vi "sub_vi_get_linear_parameters.vi"(8 "error in":errorcluster, 11 "VISA resource name in":refnum<visa-resource-name>) -> (0 "error out":errorcluster, 1 "intercept_2":dbl, 2 "slope_2":dbl, 3 "VISA resource name out":refnum<visa-resource-name>, 4 "intercept_1":dbl, 5 "slope_1":dbl, 6 "intercept_0":dbl, 7 "slope_0":dbl)   [LabVIEW 2016]
panel:
  out "result string":string
  out "read buffer":string
  out "Received values from EEPROM":dbl[](array[numeric]) format="%_6f"
  # "Slope_0"
  # "Intercept_0"
  # "Slope_1"
  # "Intercept_1"
  # "Slope_2"
  # "Intercept_2"
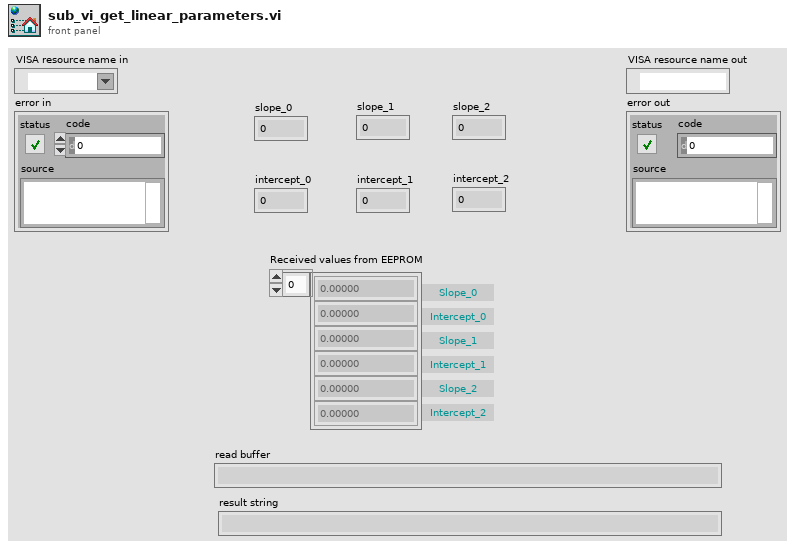
[diagram p1: front panel]
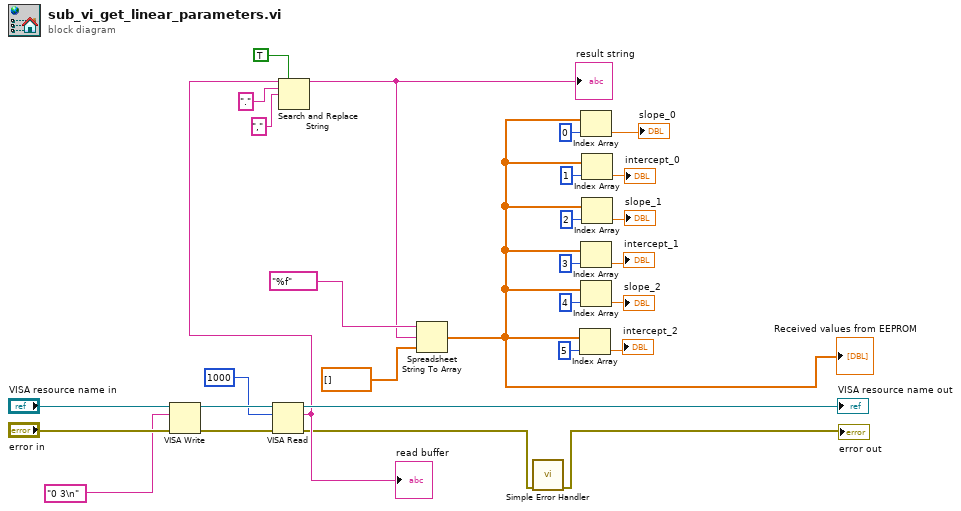
[diagram p0: block diagram]
diagram:
  n1 = VISA Write(VISA resource name="VISA resource name in", write buffer="0 3\n", error in (no error)="error in") -> (VISA resource name out=w24:refnum<visa-resource-name>, error out=w25:errorcluster)  [unwired: 1 out]
  n2 = VISA Read(VISA resource name=w24, byte count=u32 1000, error in (no error)=w25) -> (VISA resource name out=→"VISA resource name out":refnum<visa-resource-name>, read buffer=w6:string, error out=w1:errorcluster)  [unwired: 1 out]
  "read buffer" <- w6
  n3 = Search and Replace String(replace all?=TRUE ("replace all? (F)"), input string=w6, search string=".", replace string="," ("replace string (\"\")")) -> (result string=w2:string)  [unwired: 4 in, 3 out]
  "result string" <- w2
  n4 = Spreadsheet String To Array(format string="%f", spreadsheet string=w2, array type (2D Dbl)=dbl[] []) -> (array=w9:dbl[])  [unwired: 1 in]
  "Received values from EEPROM" <- w9
  n5 = call <vilib>:"Simple Error Handler.vi"("error in (no error)"=w1) -> ("error out"=→"error out":errorcluster)  [unwired: 4 in, 4 out]
  n6 = Index Array(array=w9, index=5) -> (element=→"intercept_2":dbl)
  n7 = Index Array(array=w9, index=0) -> (element=→"slope_0":dbl)
  n8 = Index Array(array=w9, index=3) -> (element=→"intercept_1":dbl)
  n9 = Index Array(array=w9, index=4) -> (element=→"slope_2":dbl)
  n10 = Index Array(array=w9, index=1) -> (element=→"intercept_0":dbl)
  n11 = Index Array(array=w9, index=2) -> (element=→"slope_1":dbl)
